vi "VI Server_STOP VI.vi"(8 "Error In":errorcluster, 11 "Path":path) -> (0 "error out":errorcluster)   [LabVIEW 2020, in "VI Server Toolkit LV2013.lvlib"]
doc: "Aborts execution of the targeted VI.\nSometimes, inadvertently, developed application gets onto infinite loop and it is impossible to stop its execution from its FP. This VI allows to interrupt the targeted VI execution without closing LabVIEW development environment."
uses:
  VI Server Toolkit LV2013.lvlib
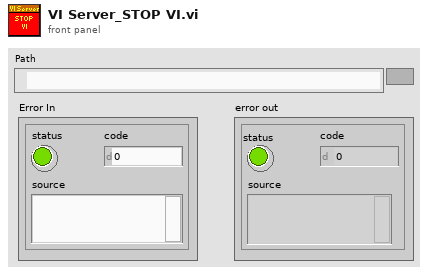
[diagram p1: front panel]
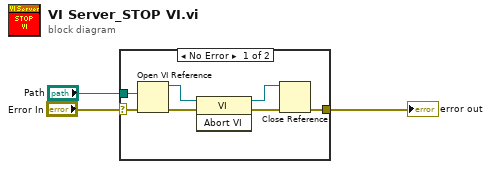
[diagram p0: block diagram]
diagram:
  n1 = case shown="No Error" "Error In" {
    selector: "Error In" -> [w4 w11]
    tunnel: "Path" -> [w10 _]
    tunnel: [w5 w11] -> w2
    frame No Error {
      n2 = Open VI Reference(vi path=w10, error in (no error)=w4) -> (vi reference=w8:refnum<vi>, error out=w9:errorcluster)  [unwired: 4 in]
      n3 = invoke class="VI" method="Abort VI"(reference=w8, error in=w9) -> (reference out=w6:refnum<vi>, error out=w7:errorcluster)  [unwired: 1 in, 1 out]
      n4 = Close Reference(reference=w6, error in (no error)=w7) -> (error out=w5:errorcluster)
    }
    frame Error {
    }
  }
  "error out" <- w2
